vi "Agilent PSG MXG Series Configure Low Frequency Output.vi"() -> ()   [LabVIEW 2018]
doc: "This example shows how to configure the low frequency output signal.\n\n<b>Note:</b>\nThis VI is valid only in N5171B, N5172B, N5181B, N5182B, N5173B, N5183B that install <B>Option UNT</B> and <B>Option 303</B> (AM, FM, phase modulation, and LF output)."
uses:
  Agilent PSG MXG Series.lvlib
panel:
  in  "Low Frequency Source (0: Monitor)":i32(ring) items=["Monitor", "Function 1", "Function 2", "Sweep", "Dual", "Noise 1", "Noise 2", "DC"]
  in  "DC Offset (0 V)":dbl
  in  "Monitor Source (0: Function 1)":i32(ring) items=["Function 1", "Function 2", "Sweep", "Dual"]
  in  "Load Impedance (50: 50 Ohm)":i32(ring)=50 items=["50 Ohm"=50, "1000000 Ohm"=1000000]
  in  "Low Frequency Output Amplitude (1)":dbl=1.0
  in  "Tone Path (1: 1)":i32(ring)=1 items=["1"=1, "2"=2]
  in  "Frequency (400 Hz)":dbl=400.0
  in  "Modulation Path (1: 1)":i32(ring)=1 items=["1"=1, "2"=2]
  in  "Waveform Type (0: Sine)":i32(ring) items=["Sine", "Triangle", "Square", "Ramp", "Pulse", "Noise", "DC"]
  in  "VISA resource name":refnum<visa-resource-name>
  # "(c) 2007-2016 National Instruments.  ALL RIGHTS RESERVED."
  # "This VI is valid only in N5171B, N5172B, N5181B, N5182B, N5173B, \nN5183B that install Option UNT and Option 303."
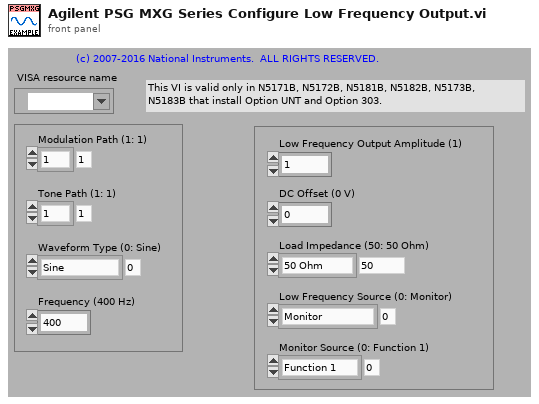
[diagram p1: front panel]
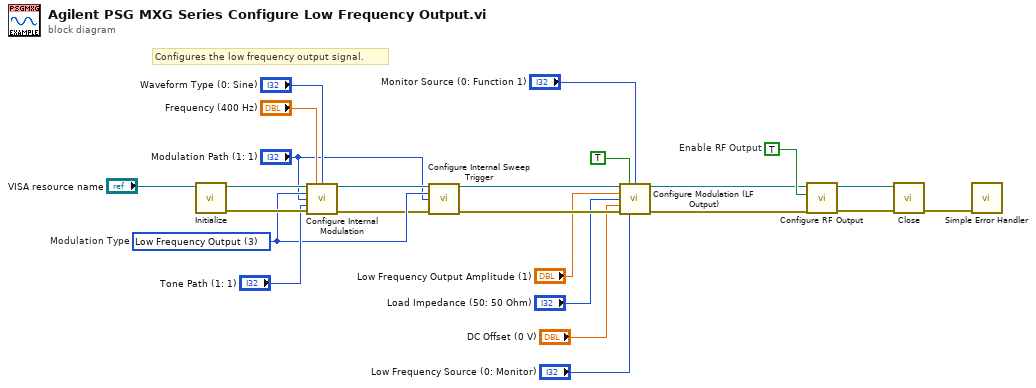
[diagram p0: block diagram]
diagram:
  w14 = 3 items=["Amplitude Modulation", "Frequency Modulation", "Phase Modulation", "Low Frequency Output"]  # Modulation Type
  w20 = TRUE  # Enable RF Output
  # "Configures the low frequency output signal."
  n1 = call "Initialize.vi"("VISA resource name"="VISA resource name") -> ("error out"=w17:errorcluster, "VISA resource name out"=w18:refnum<visa-resource-name>)  [unwired: 3 in, 6 out]
  n2 = call "Configure Internal Modulation.vi"("VISA resource name"=w18, "Frequency (400 Hz)"="Frequency (400 Hz)", "Waveform Type (0: Sine)"="Waveform Type (0: Sine)", "Modulation Type (0: Amplitude Modulation)"=w14, "Modulation Path (1: 1)"="Modulation Path (1: 1)", "Tone Path (1: 1)"="Tone Path (1: 1)", "error in (no error)"=w17) -> ("VISA resource name out"=w12:refnum<visa-resource-name>, "error out"=w13:errorcluster)  [unwired: 2 in, 5 out]
  n3 = call "Configure Internal Sweep Trigger.vi"("VISA resource name"=w12, "Modulation Type (0: Amplitude Modulation)"=w14, "Modulation Path (1: 1)"="Modulation Path (1: 1)", "error in (no error)"=w13) -> ("VISA resource name out"=w10:refnum<visa-resource-name>, "error out"=w9:errorcluster)  [unwired: 4 in, 6 out]
  n4 = call "Configure Modulation (LF Output).vi"("VISA resource name"=w10, "Enable Low Frequency Output (F: Disable)"=TRUE, "Monitor Source (0: Function 1)"="Monitor Source (0: Function 1)", "Low Frequency Output Amplitude (0 VP)"="Low Frequency Output Amplitude (1)", "Load Impedance (50: 50 Ohm)"="Load Impedance (50: 50 Ohm)", "DC Offset (0 V)"="DC Offset (0 V)", "error in (no error)"=w9, "Low Frequency Source (0: Monitor)"="Low Frequency Source (0: Monitor)") -> ("VISA resource name out"=w2:refnum<visa-resource-name>, "error out"=w1:errorcluster)  [unwired: 6 out]
  n5 = call "Configure RF Output.vi"("error in (no error)"=w1, "Enable RF Output (F:Disable)"=w20, "VISA resource name"=w2) -> ("error out"=w22:errorcluster, "VISA resource name out"=w23:refnum<visa-resource-name>)  [unwired: 5 in, 2 out]
  n6 = call "Close.vi"("error in (no error)"=w22, "VISA resource name"=w23) -> ("error out"=w24:errorcluster)  [unwired: 9 out]
  n7 = call <vilib>:"Simple Error Handler.vi"("error in (no error)"=w24) -> ()  [unwired: 1 in, 8 out]
